vi "Export - Buffered Tx Packet.vi"(8 "error in (no error)":errorcluster, 11 "Device Item Ref in":T6 format="%.0x") -> (0 "error out":errorcluster, 3 "Tx Packet":T1 {"Endianness" items=["big-endian"=0, "little-endian"=2]})   [LabVIEW 2016, in "UDP-Custom-Device System Explorer.lvlib"]
uses:
  UDP-Custom-Device System Explorer.lvlib
  <vilib>/NI Veristand/Custom Device API/Custom Device Item Ref.ctl
  Types/XML - New/ImpExp - Tx Packet Data.ctl
  <vilib>/NI Veristand/Custom Device API/Custom Device Item Info.ctl
  Shared/Types/Shared - Channel Data Type.ctl
  Shared/Types/Shared - Buffered.PacketInfo.ctl
  Shared/Types/Shared - Pointer Encoding.ctl
  Property Accessors/Shared Packet Accessors.lvlib
  Property Accessors/Tx Packet Accessors.lvlib
  <vilib>/NI VeriStand/Custom Device API/Custom Device API.lvlib
  Shared/UDP-Custom-Device Shared.lvlib
  <vilib>/NI VeriStand/Custom Device Tools/Custom Device Utility Library/Custom Device Utility Library.lvlib
  Property Accessors/Buffered Data Packet.lvlib
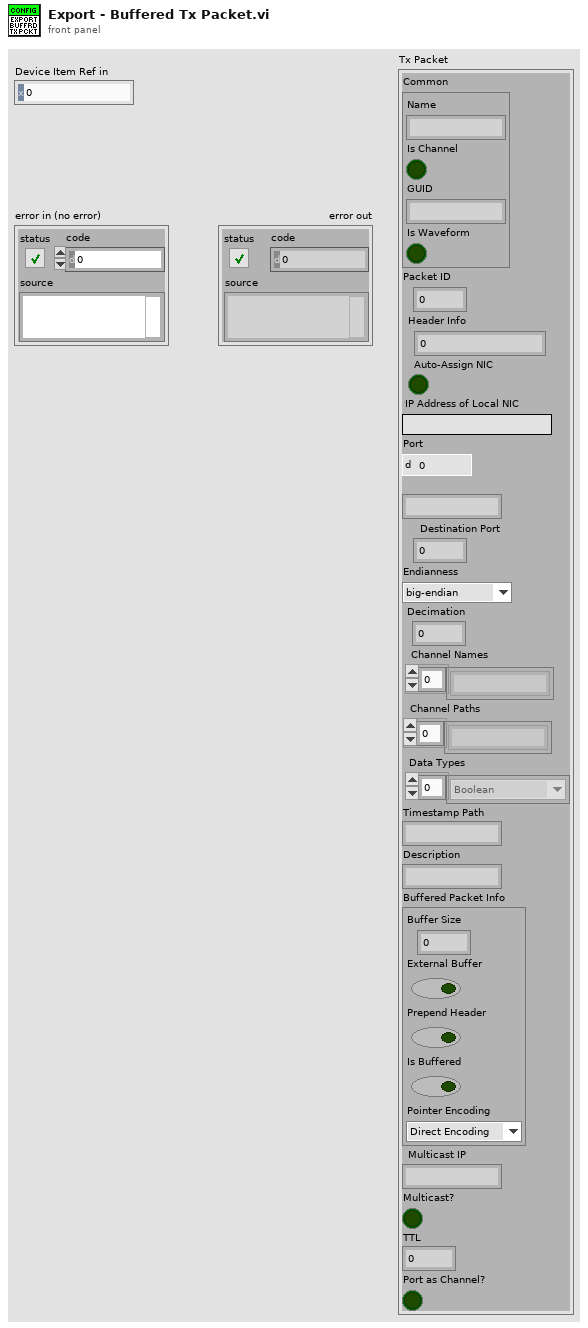
[diagram p1: front panel]
types:
  T1 = typedef "UDP-Custom-Device System Explorer.lvlib/ImpExp - Tx Packet Data.ctl" = cluster{"Common":T2, "Packet ID":i32, "Header Info":u32, "Auto-Assign NIC":bool, "IP Address of Local NIC":string, "Port":u16, "Destination IP":string, "Destination Port":u16, "Endianness":u16, "Decimation":u16, "Channel Names":string[], "Channel Paths":string[], "Data Types":T3[], "Timestamp Path":string, "Description":string, "Buffered Packet Info":T4, "Multicast IP":string, "Multicast?":bool, "TTL":u16, "Port as Channel?":bool}
  T2 = typedef "Custom Device API.lvlib/Custom Device Item Info.ctl" = cluster{"Name":string, "Is Channel":bool, "GUID":string, "Is Waveform":bool}
  T3 = typedef "UDP-Custom-Device Shared.lvlib/Shared - Channel Data Type.ctl" = enum16{"Boolean", "Single", "Double", "I8", "I16", "I32", "I64", "U8", "U16", "U32", "U64"}
  T4 = typedef "UDP-Custom-Device Shared.lvlib/Shared - Buffered.PacketInfo.ctl" = cluster{"Buffer Size":i32, "External Buffer":bool, "Prepend Header":bool, "Is Buffered":bool, "Pointer Encoding":T5}
  T5 = typedef "UDP-Custom-Device Shared.lvlib/Shared - Pointer Encoding.ctl" = enum16{"Direct Encoding", "Conversion Encoding"}
  T6 = typedef "Custom Device API.lvlib/Custom Device Item Ref.ctl" = u64
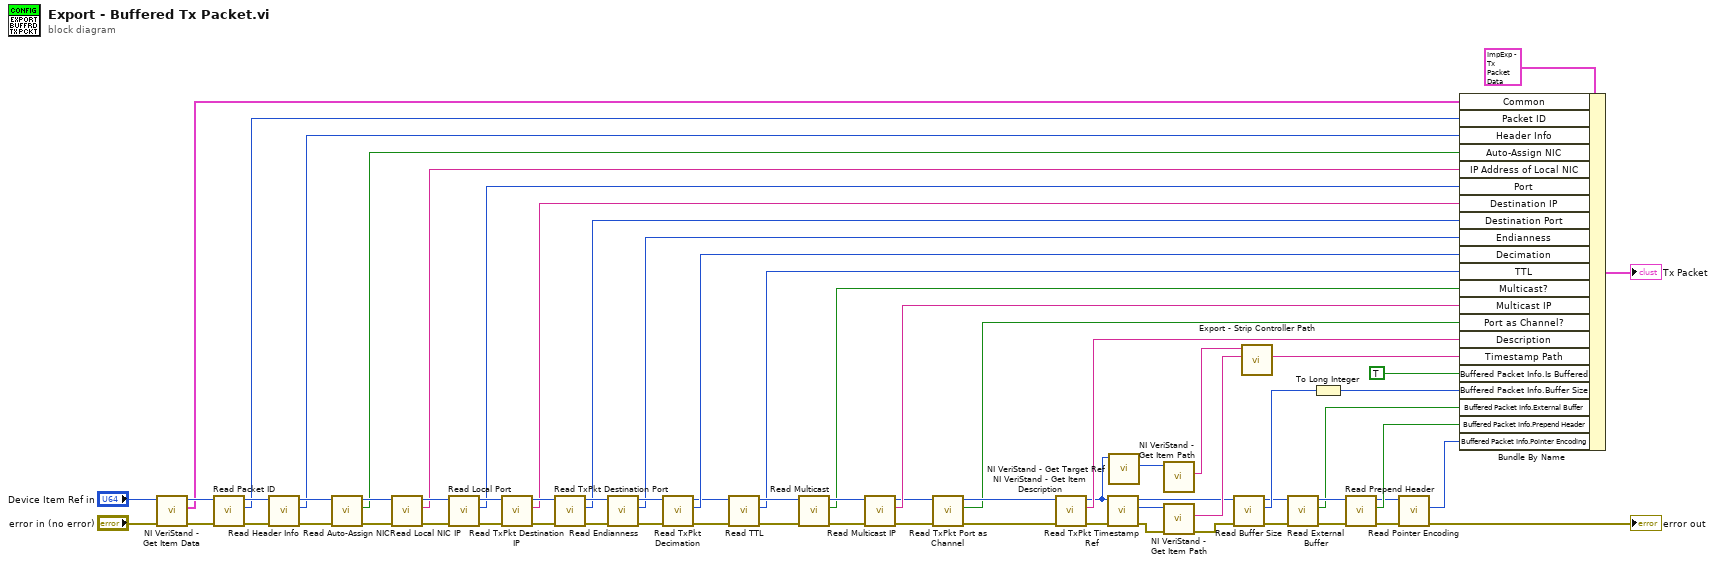
[diagram p0: block diagram]
diagram:
  n1 = call <vilib>:"NI VeriStand - Get Item Data.vi"("error in (no error)"="error in (no error)", "Item Ref in"="Device Item Ref in") -> ("error out"=w70:errorcluster, "Item Info"=w48:T2, "Item Ref out"=w53:T6)  [unwired: 6 in, 1 out]
  n2 = call "Read Packet ID.vi"("error in (no error)"=w70, "Node Ptr"=w53) -> ("error out"=w55:errorcluster, "Packet ID"=w47:i32, "Node Ptr out"=w54:T6)  [unwired: 7 in]
  n3 = call "Read Header Info.vi"("error in (no error)"=w55, "Node Ptr"=w54) -> ("error out"=w57:errorcluster, "Header Info"=w46:u32, "Node Ptr out"=w56:T6)  [unwired: 7 in]
  n4 = call "Read Auto-Assign NIC.vi"("error in (no error)"=w57, "Node Ptr"=w56) -> ("error out"=w61:errorcluster, "Auto-Assign NIC"=w45:bool, "Node Ptr out"=w58:T6)  [unwired: 7 in]
  n5 = call "Read Local NIC IP.vi"("error in (no error)"=w61, "Node Ptr"=w58) -> ("error out"=w60:errorcluster, "IP Address of Local NIC"=w44:string, "Node Ptr out"=w59:T6)  [unwired: 7 in]
  n6 = call "Read Local Port.vi"("error in (no error)"=w60, "Node Ptr"=w59) -> ("error out"=w63:errorcluster, "Port"=w43:u16, "Node Ptr out"=w62:T6)  [unwired: 7 in]
  n7 = call "Read TxPkt Destination IP.vi"("error in (no error)"=w63, "Node Ptr"=w62) -> ("error out"=w65:errorcluster, "Destination IP"=w42:string, "Node Ptr out"=w64:T6)  [unwired: 7 in]
  n8 = call "Read TxPkt Destination Port.vi"("error in (no error)"=w65, "Node Ptr"=w64) -> ("error out"=w67:errorcluster, "Destination Port"=w41:u16, "Node Ptr out"=w66:T6)  [unwired: 7 in]
  n9 = call "Read Endianness.vi"("error in (no error)"=w67, "Node Ptr"=w66) -> ("error out"=w69:errorcluster, "Endianness"=w40:u16, "Node Ptr out"=w68:T6)  [unwired: 7 in]
  n10 = call "Read TxPkt Decimation.vi"("error in (no error)"=w69, "Node Ptr"=w68) -> ("error out"=w13:errorcluster, "Decimation"=w39:u16, "Node Ptr out"=w16:T6)  [unwired: 7 in]
  n11 = call "Read TTL.vi"("error in (no error)"=w13, "Node Ptr"=w16) -> ("error out"=w14:errorcluster, "TTL"=w12:u16, "Node Ptr out"=w18:T6)  [unwired: 7 in]
  n12 = call "Read Multicast.vi"("error in (no error)"=w14, "Node Ptr"=w18) -> ("error out"=w15:errorcluster, "Multicast"=w11:bool, "Node Ptr out"=w17:T6)  [unwired: 7 in]
  n13 = call "Read Multicast IP.vi"("error in (no error)"=w15, "Node Ptr"=w17) -> ("error out"=w3:errorcluster, "Multicast IP Address"=w10:string, "Node Ptr out"=w5:T6)  [unwired: 7 in]
  n14 = call "Read TxPkt Port as Channel.vi"("error in (no error)"=w3, "Node Ptr"=w5) -> ("error out"=w2:errorcluster, "Port as Channel"=w1:bool, "Node Ptr out"=w4:T6)  [unwired: 7 in]
  n15 = call <vilib>:"NI VeriStand - Get Item Description.vi"("error in (no error)"=w2, "Item Ref in"=w4) -> ("error out"=w35:errorcluster, "Description"=w38:string, "Item Ref out"=w31:T6)  [unwired: 6 in, 1 out]
  n16 = call "Read TxPkt Timestamp Ref.vi"("error in (no error)"=w35, "Node Ptr"=w31) -> ("error out"=w34:errorcluster, "Timestamp Ref"=w36:T6, "Node Ptr out"=w23:T6)  [unwired: 7 in]
  n17 = call <vilib>:"NI VeriStand - Get Target Ref.vi"("Item Ref in"=w31) -> ("Target Ref"=w32:T6)  [unwired: 7 in, 3 out]
  n18 = call <vilib>:"NI VeriStand - Get Item Path.vi"("Item Ref in"=w32) -> ("Path"=w30:string)  [unwired: 7 in, 3 out]
  n19 = call <vilib>:"NI VeriStand - Get Item Path.vi"("error in (no error)"=w34, "Item Ref in"=w36) -> ("error out"=w22:errorcluster, "Path"=w37:string)  [unwired: 6 in, 2 out]
  n20 = call "Read Buffer Size.vi"("error in (no error)"=w22, "Node Ptr"=w23) -> ("error out"=w26:errorcluster, "Buffer Size"=w28:u32, "Node Ptr out"=w24:T6)  [unwired: 7 in]
  n21 = call "Export - Strip Controller Path.vi"("Channel Path"=w37, "Controller Path"=w30) -> ("Stripped Path"=w33:string)  [unwired: 8 in, 1 out]
  n22 = call "Read External Buffer.vi"("error in (no error)"=w26, "Node Ptr"=w24) -> ("error out"=w27:errorcluster, "External Buffer"=w20:bool, "Node Ptr out"=w25:T6)  [unwired: 7 in]
  n23 = To Long Integer(number=w28) -> (32bit integer=w21:i32)
  n24 = call "Read Prepend Header.vi"("error in (no error)"=w27, "Node Ptr"=w25) -> ("error out"=w8:errorcluster, "Prepend Header"=w19:bool, "Node Ptr out"=w9:T6)  [unwired: 7 in]
  n25 = call "Read Pointer Encoding.vi"("error in (no error)"=w8, "Node Ptr"=w9) -> ("error out"=→"error out":errorcluster, "Pointer Encoding"=w6:T5)  [unwired: 7 in, 1 out]
  n26 = Bundle By Name(cluster=T1 {"Common"={"Name"="", "Is Channel"=FALSE, "GUID"="", "Is Waveform"=FALSE}, "Packet ID"=0, "Header Info"=0, "Auto-Assign NIC"=FALSE, "IP Address of Local NIC"="", "Port"=0, "Destination IP"="", "Destination Port"=0, "Endianness"=0, "Decimation"=0, "Channel Names"=[], "Channel Paths"=[], "Data Types"=[], "Timestamp Path"="", "Description"="", "Buffered Packet Info"={"Buffer Size"=0, "External Buffer"=FALSE, "Prepend Header"=FALSE, "Is Buffered"=FALSE, "Pointer Encoding"=enum."Direct Encoding"}, "Multicast IP"="", "Multicast?"=FALSE, "TTL"=0, "Port as Channel?"=FALSE} ("Tx Packet"), "Common"=w48, "Packet ID"=w47, "Header Info"=w46, "Auto-Assign NIC"=w45, "IP Address of Local NIC"=w44, "Port"=w43, "Destination IP"=w42, "Destination Port"=w41, "Endianness"=w40, "Decimation"=w39, "TTL"=w12, "Multicast?"=w11, "Multicast IP"=w10, "Port as Channel?"=w1, "Description"=w38, "Timestamp Path"=w33, "Buffered Packet Info.Is Buffered"=TRUE, "Buffered Packet Info.Buffer Size"=w21, "Buffered Packet Info.External Buffer"=w20, "Buffered Packet Info.Prepend Header"=w19, "Buffered Packet Info.Pointer Encoding"=w6) -> (→"Tx Packet":T1)
